vi "fg_ROI Management.vi"(5 "Function":T4, 8 "error in (no error)":errorcluster, 9 "ROI management Input cluster":T2, 10 "Offsets cluster":T1, 11 "Reuse last composite ID":bool) -> (0 "error out":errorcluster, 1 "Last composite ID":i32, 2 "Number of ROI":i32, 3 "ROI Setup":T5[](array[typedef]) {"ROI group ID" format="%#_6f"; "Laser Power (%)" format="%#_6f"; "Zoom" format="%#_6f"; "Frame Size" format="%#_6f"; "Number of lines" format="%#_6f"; "Composite ID" format="%#_6f"; "Angle (deg)" format="%#_6f"; "ROI Time (ns)" format="%#_6f"; "ROI ID" format="%#_6f"; "Pixels in ROI" format="%#_6f"; "ROI index" format="%#_6f"; "Z stop" format="%#_6f"; "Y stop" format="%#_6f"; "X stop" format="%#_6f"; "Z start" format="%#_6f"; "X start" format="%#_6f"; "Y start" format="%#_6f"}, 6 "Exceeded limit number of lines":bool)   [LabVIEW 2013]
uses:
  Visualisation/Functional Imaging Viewer/Typedefs/ROI parameters data type.ctl
  Typedefs/ROI management FG states.ctl
  Typedefs/ROI management Input cluster.ctl
  Typedefs/ROI ID Enum.ctl
  Typedefs/Offsets cluster.ctl
  Global Variables/General Globals.vi
  ROI Entry screen/Globals/gl_ROI Entry UI globals.vi
panel:
  out "Number of lines left":i32
  # "X Start\nY Start\nX Stop\nY Stop"
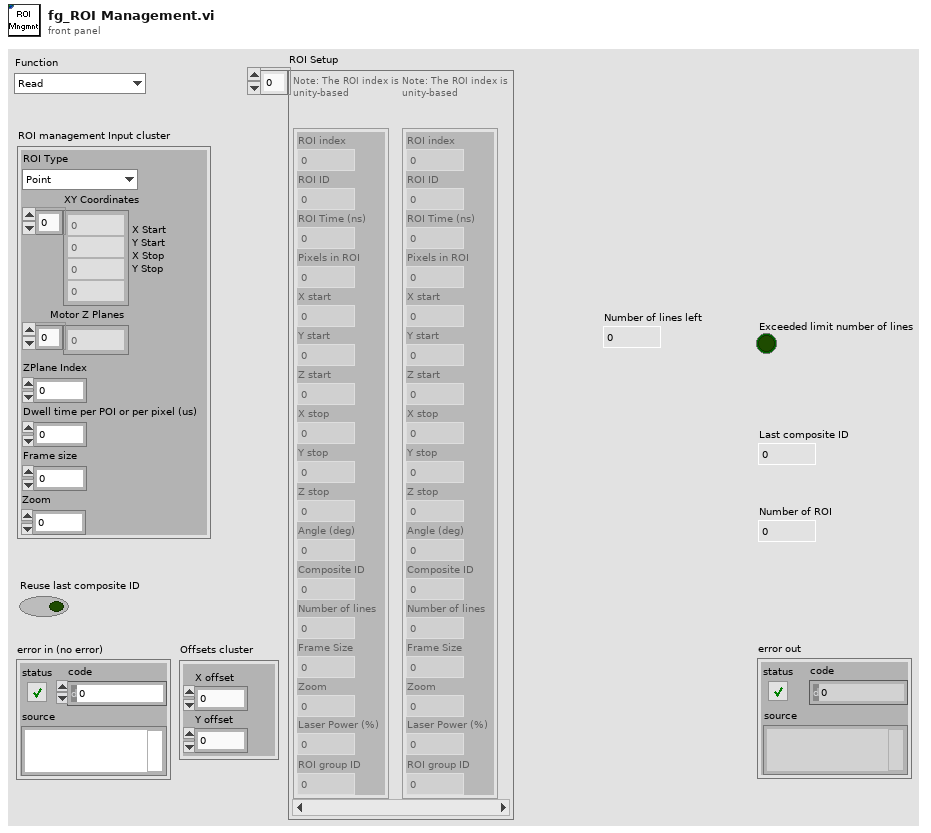
[diagram p1: front panel]
types:
  T1 = typedef "Offsets cluster.ctl" = cluster{"X offset":i8, "Y offset":i8}
  T2 = typedef "ROI management Input cluster.ctl" = cluster{"ROI Type":T3, "XY Coordinates":i32[], "Motor Z Planes":dbl[], "ZPlane Index":i32, "Dwell time per POI or per pixel (us)":dbl, "Frame size":i32, "Zoom":dbl}
  T3 = typedef "ROI ID Enum.ctl" = enum16{"Point", "MiniScan", "Comp. MiniScan", "Rectangle", "Comp. volume", "Arb. plane point"}
  T4 = typedef "ROI management FG states.ctl" = enum16{"Read", "Write", "Clear Last", "Clear All", "Update ROIs time", "Reload last ROI set", "Offset all ROI", "Offset visible ROI"}
  T5 = typedef "ROI parameters data type.ctl" = cluster{"ROI index":dbl, "ROI ID":dbl, "ROI Time (ns)":dbl, "Pixels in ROI":dbl, "X start":dbl, "Y start":dbl, "Z start":dbl, "X stop":dbl, "Y stop":dbl, "Z stop":dbl, "Angle (deg)":dbl, "Composite ID":dbl, "Number of lines":dbl, "Frame Size":dbl, "Zoom":dbl, "Laser Power (%)":dbl, "ROI group ID":dbl}
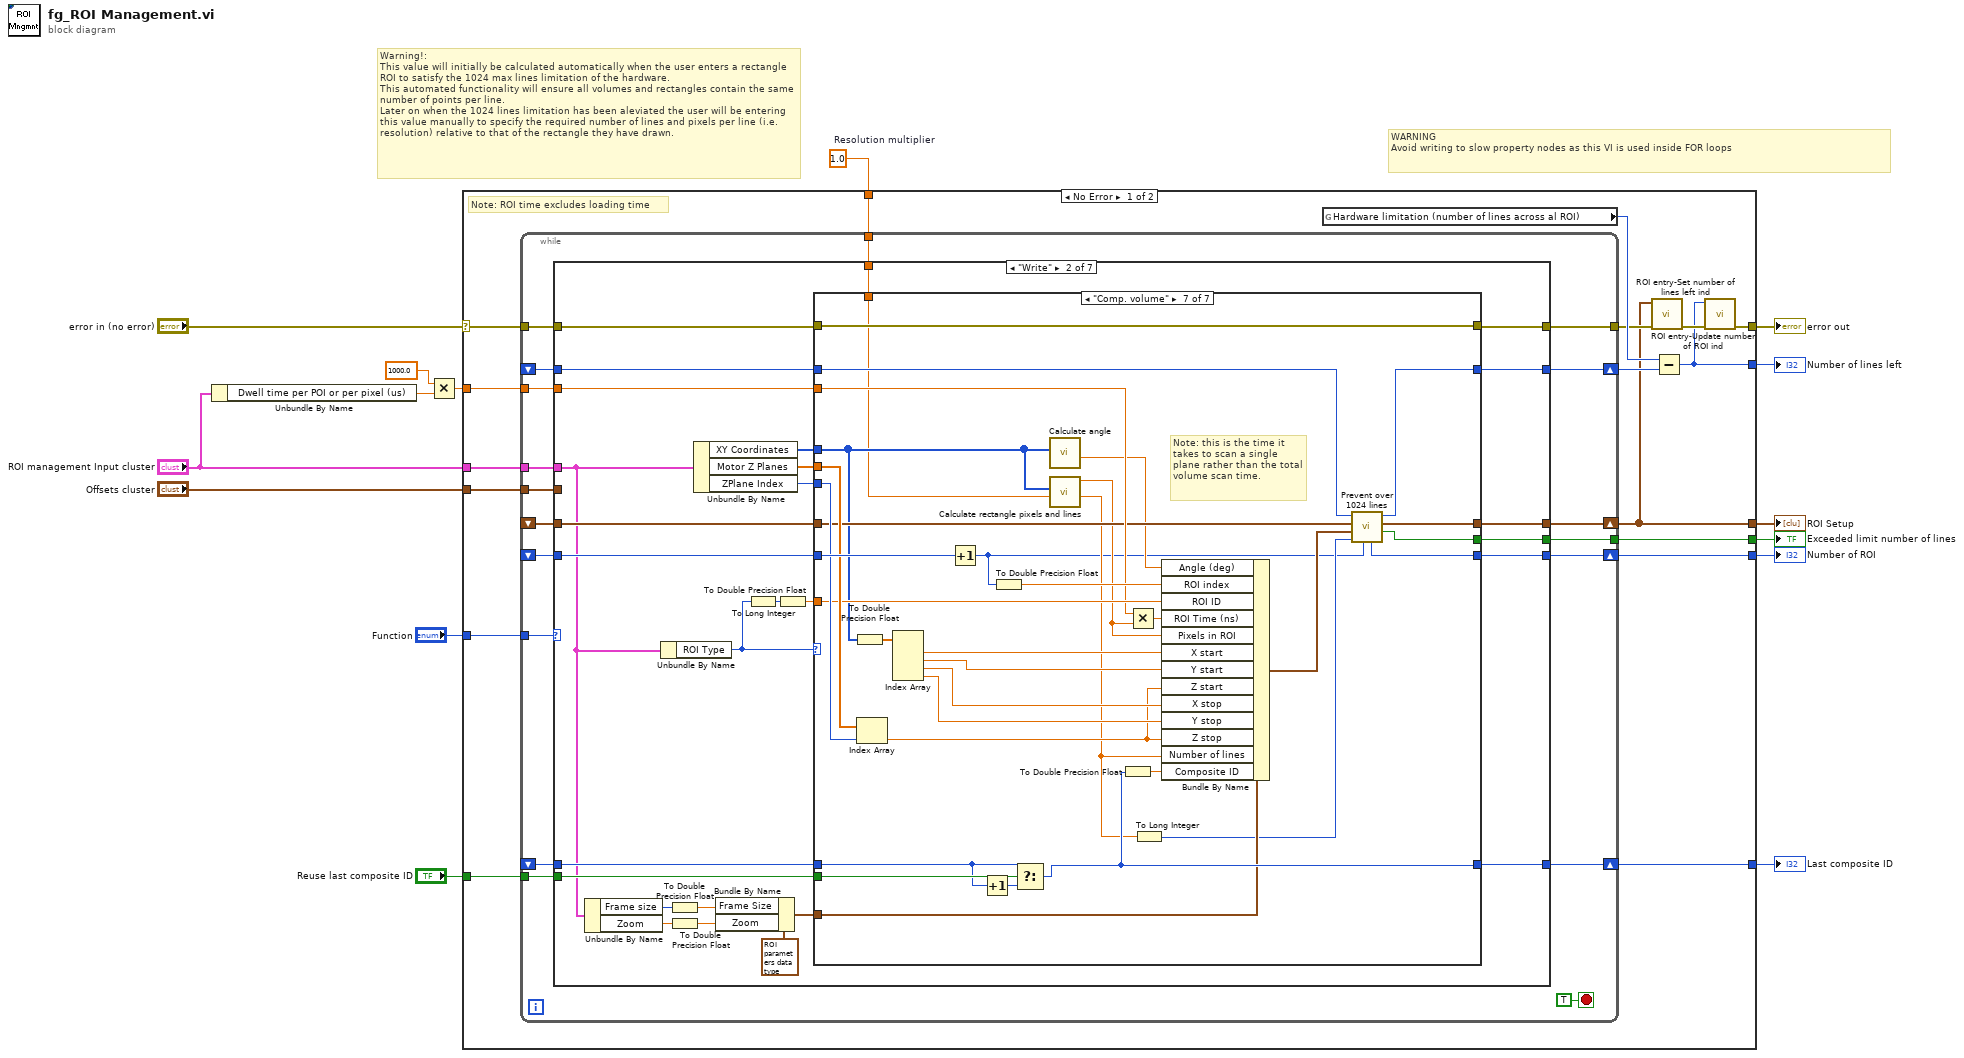
[diagram p0: block diagram]
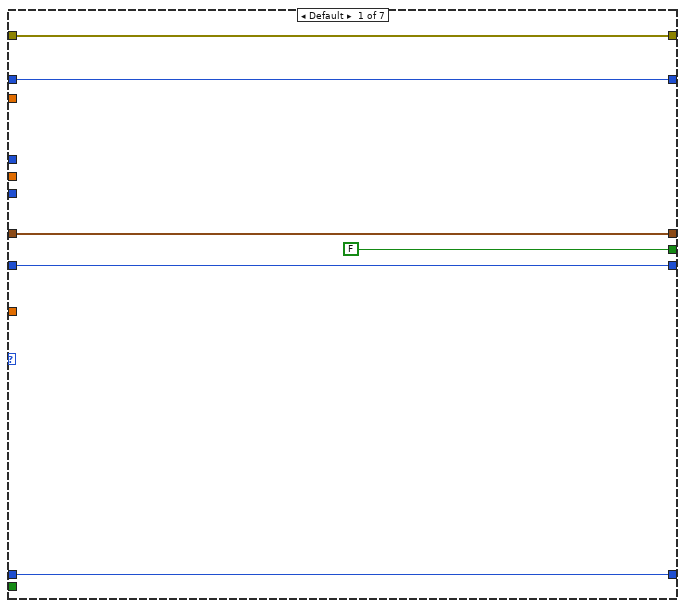
[diagram p3: hidden frame]
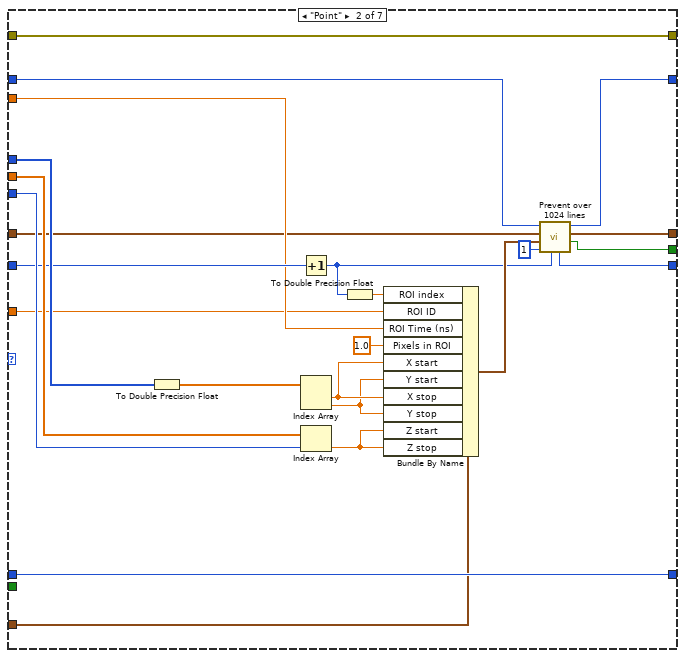
[diagram p4: hidden frame]
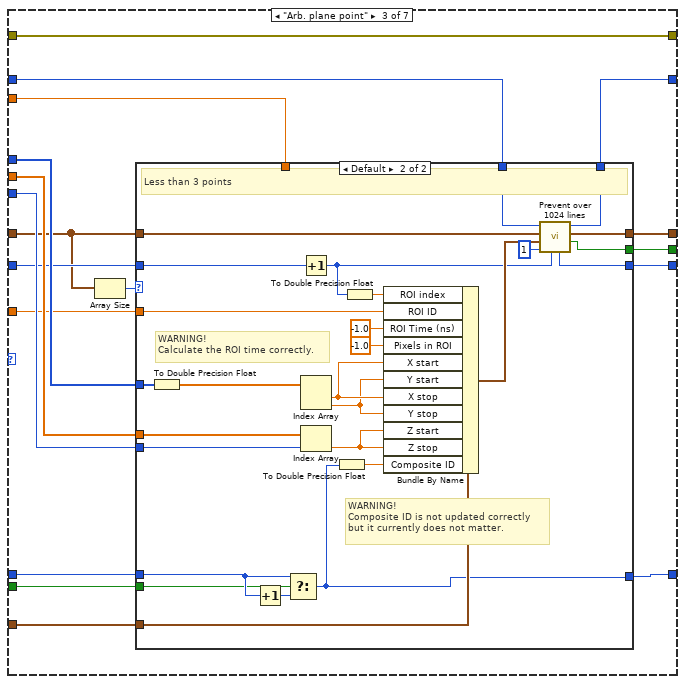
[diagram p5: hidden frame]
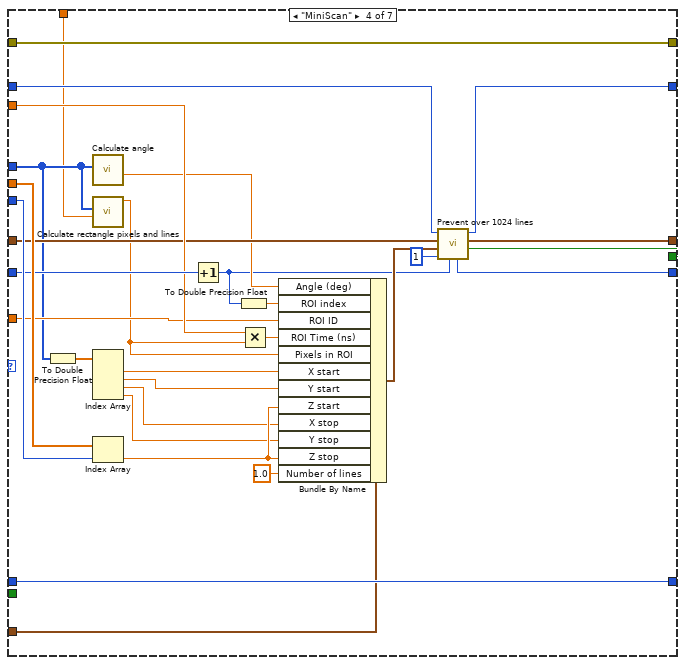
[diagram p7: hidden frame]
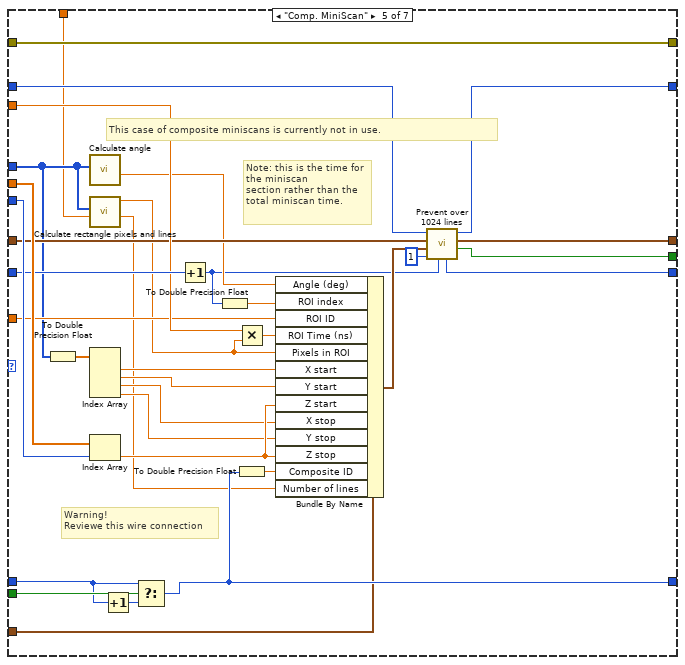
[diagram p8: hidden frame]
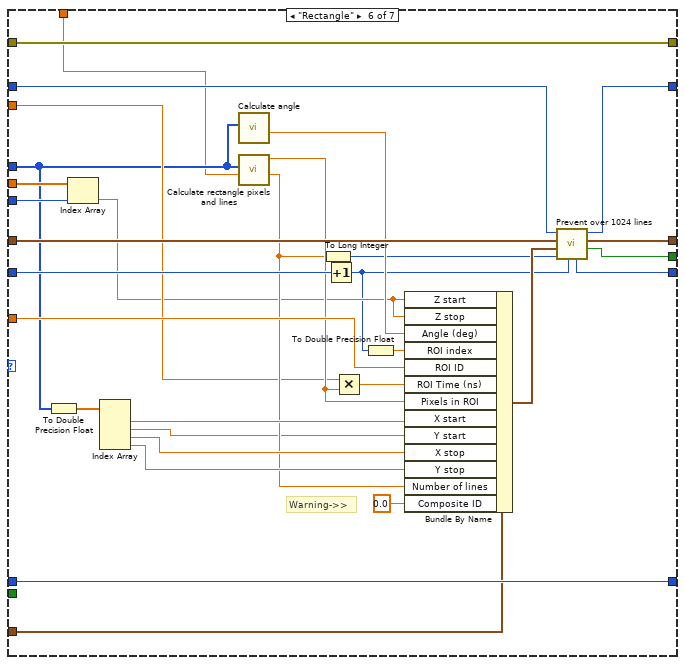
[diagram p9: hidden frame]
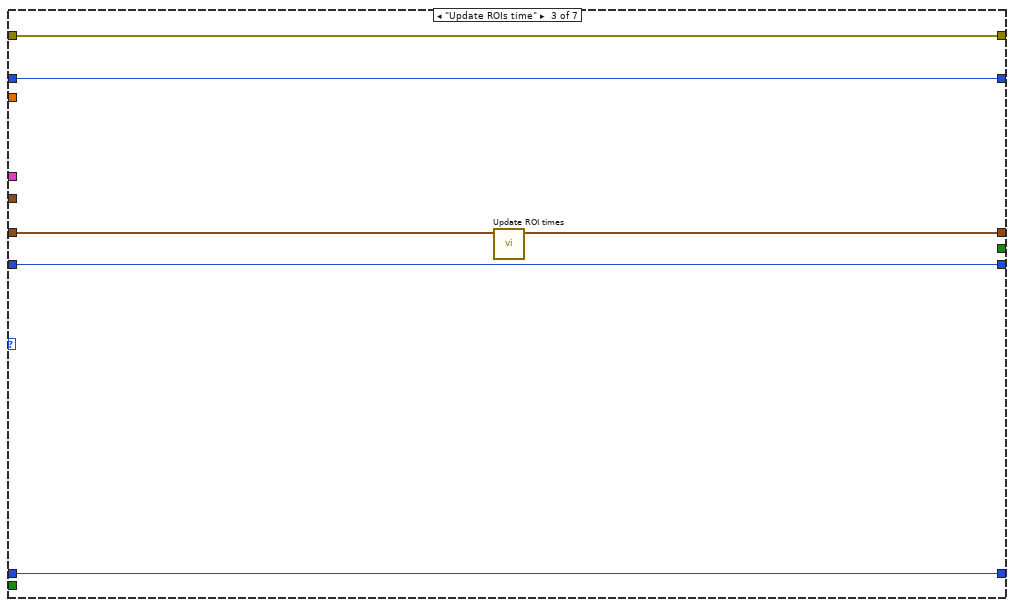
[diagram p10: hidden frame]
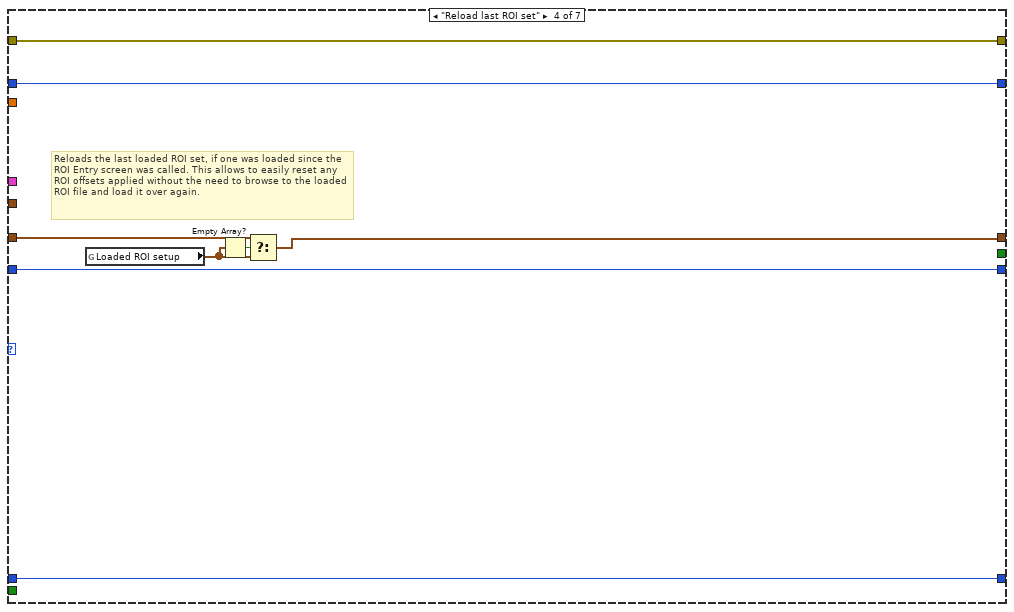
[diagram p11: hidden frame]
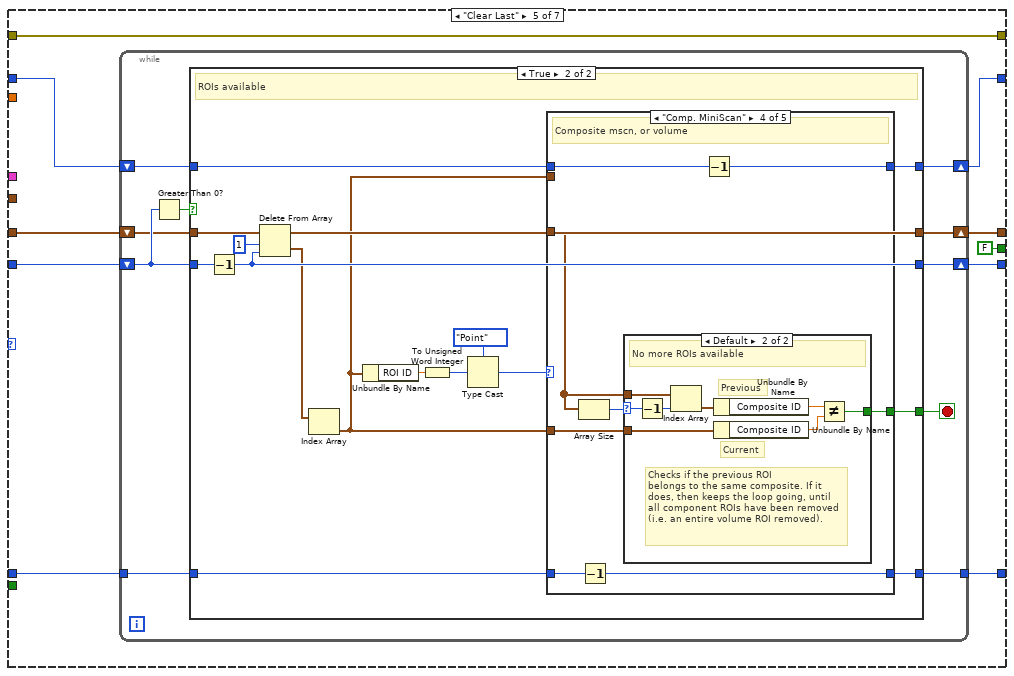
[diagram p12: hidden frame]
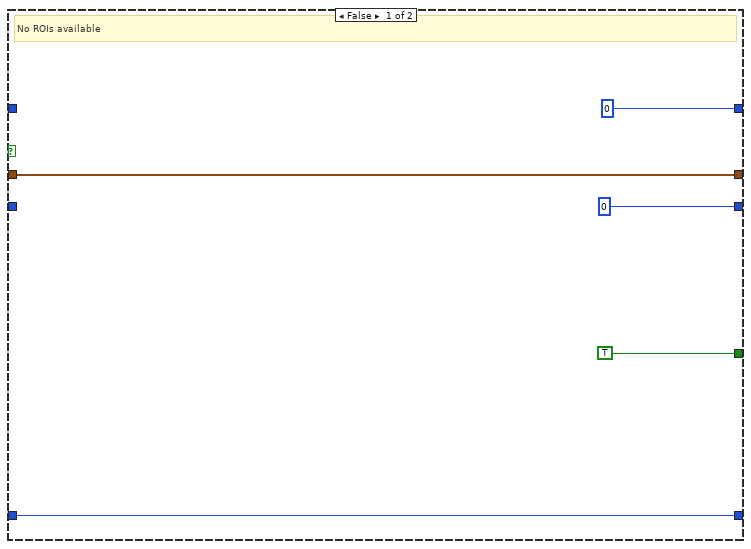
[diagram p13: hidden frame]
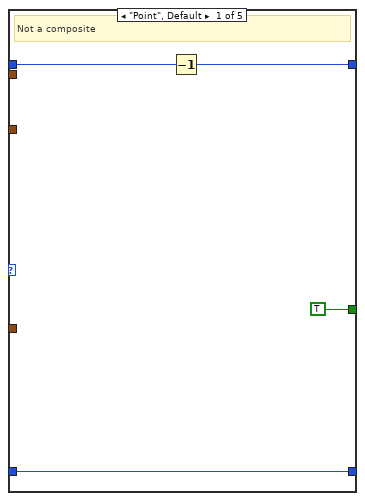
[diagram p14: hidden frame]
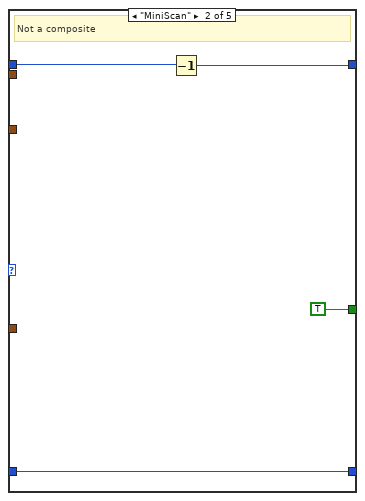
[diagram p15: hidden frame]
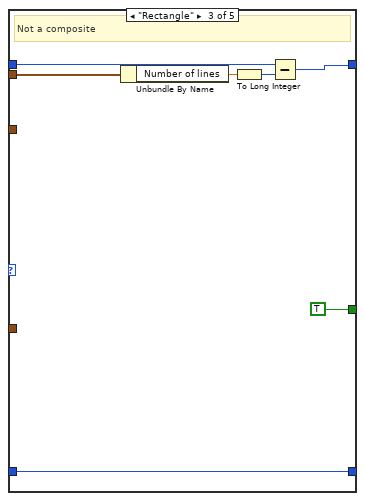
[diagram p16: hidden frame]
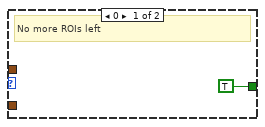
[diagram p17: hidden frame]
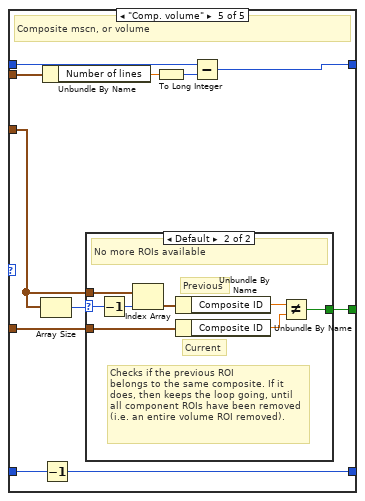
[diagram p18: hidden frame]
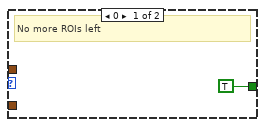
[diagram p19: hidden frame]
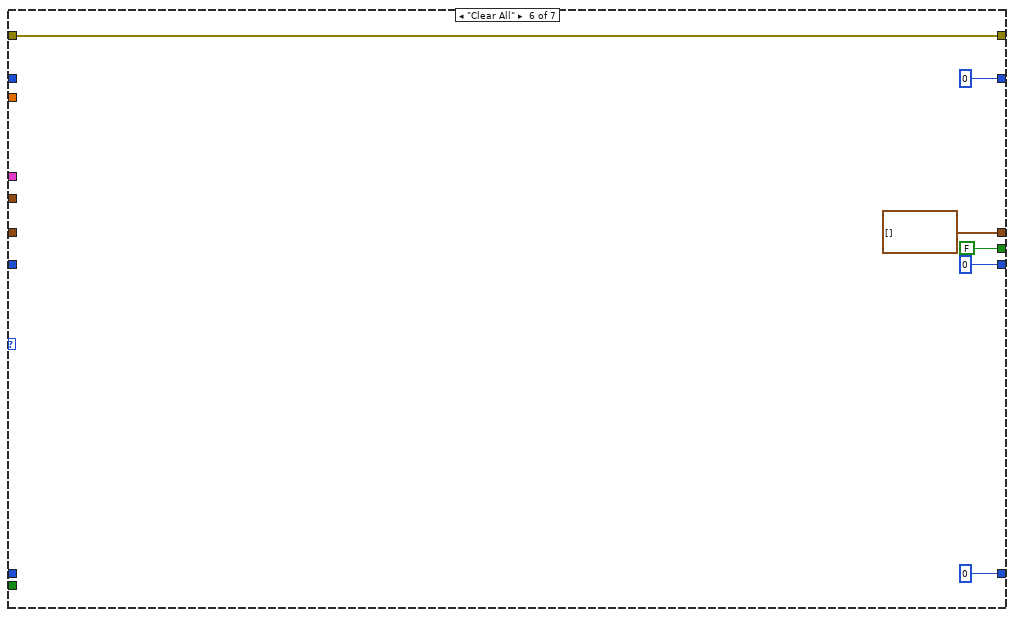
[diagram p20: hidden frame]
diagram:
  w5 = 1.0  # Resolution multiplier
  # "WARNING\nAvoid writing to slow property nodes as this VI is used inside FOR loops"
  # "Warning!:\nThis value will initially be calculated automatically when the user enters a rectangle ROI to satisfy the 1024 max lines limitation of the hardware.\nThis automated functionality will ensure all volumes and rectangles contain the same number of points per line.\nLater on when the 1024 lines limitation has been aleviated the user will be entering this value manually to specify the required number of lines and pixels per line (i.e. resolution) relative to that of the rectangle they have drawn."
  n1 = Unbundle By Name("ROI management Input cluster") -> ("Dwell time per POI or per pixel (us)"=w6:dbl)
  n2 = Multiply(x=1000.0, y=w6) -> (x*y=w11:dbl)
  n3 = case shown="No Error" "error in (no error)" {
    selector: "error in (no error)" -> [w32 w412]
    tunnel: [w18 w412] -> w12
    tunnel: [w20 _] -> w14
    tunnel: w11 -> [w31 _]
    tunnel: "Function" -> [w30 _]
    tunnel: [w29 _] -> w9
    tunnel: [w28 _] -> w8
    tunnel: "Reuse last composite ID" -> [w27 _]
    tunnel: "ROI management Input cluster" -> [w26 _]
    tunnel: w5 -> [w25 _]
    tunnel: [w17 _] -> w3
    tunnel: [w22 _] -> w2
    tunnel: "Offsets cluster" -> [w16 _]
    frame No Error {
      # "Note: ROI time excludes loading time"
      n4 = while {
        tunnel: w32 -> [w50]
        tunnel: [w49] -> w21
        shift-right: [w48] -> w20
        shift-left: _ -> [w46]
        tunnel: w31 -> [w47]
        shift-right: [w45] -> w29
        shift-left: _ -> [w44]
        tunnel: w30 -> [w43]
        shift-right: [w40] -> w28
        shift-left: _ -> [w41]
        tunnel: w27 -> [w39]
        tunnel: w26 -> [w38]
        shift-right: [w37] -> w24
        shift-left: _ -> [w36]
        tunnel: w25 -> [w35]
        tunnel: [w34] -> w22
        tunnel: w16 -> [w33]
        stop <- TRUE stop-if-true
        n5 = case shown="\"Write\"" w43 {
          selector: w43 -> [_ _ _ _ _ _ w404]
          tunnel: w50 -> [w53 w82 w294 w303 w312 w402 w410]
          tunnel: [w53 w81 w294 w303 w312 w402 w410] -> w49
          tunnel: [w55 w80 w296 w298 w313 T5[] [] w405] -> w48
          tunnel: w47 -> [_ w79 _ _ _ _ _]
          tunnel: w46 -> [w55 w78 w292 w299 w308 _ w408]
          tunnel: [w54 w77 w295 w304 w314 0 w411] -> w45
          tunnel: w44 -> [w54 w76 w295 w304 w309 _ w411]
          tunnel: w41 -> [w52 w72 w291 w301 w311 _ w407]
          tunnel: [w52 w73 w291 w301 w310 0 ("Last composite ID") w407] -> w40
          tunnel: w39 -> [_ w71 _ _ _ _ _]
          tunnel: w38 -> [_ w65 _ _ _ _ _]
          tunnel: [w51 w58 w293 w302 w305 0 w409] -> w37
          tunnel: w36 -> [w51 w60 w293 w302 w307 _ w409]
          tunnel: w35 -> [_ w59 _ _ _ _ _]
          tunnel: [_ w57 _ _ FALSE ("Exceeded 1024 lines") FALSE ("Exceeded 1024 lines") _] -> w34
          tunnel: w33 -> [_ _ _ _ _ _ w406]
          frame "Read", Default {
          }
          frame "Write" {
            n6 = Unbundle By Name(w65) -> ("Frame size"=w66:i32, "Zoom"=w62:dbl)
            n7 = Unbundle By Name(w65) -> ("ROI Type"=w67:T3)
            n8 = To Double Precision Float(number=w66) -> (double precision float=w64:dbl)
            n9 = To Double Precision Float(number=w62) -> (double precision float=w61:dbl)
            n10 = Unbundle By Name(w65) -> ("XY Coordinates"=w70:i32[], "Motor Z Planes"=w69:dbl[], "ZPlane Index"=w68:i32)
            n11 = Bundle By Name(cluster=T5 {"ROI index"=0.0, "ROI ID"=0.0, "ROI Time (ns)"=0.0, "Pixels in ROI"=0.0, "X start"=0.0, "Y start"=0.0, "Z start"=0.0, "X stop"=0.0, "Y stop"=0.0, "Z stop"=0.0, "Angle (deg)"=0.0, "Composite ID"=0.0, "Number of lines"=0.0, "Frame Size"=0.0, "Zoom"=0.0, "Laser Power (%)"=0.0, "ROI group ID"=0.0} ("X-Y-Z coordinates"), "Frame Size"=w64, "Zoom"=w61) -> (w63:T5)
            n12 = To Long Integer(number=w67) -> (32bit integer=w75:i32)
            n13 = To Double Precision Float(number=w75) -> (double precision float=w74:dbl)
            n14 = case shown="\"Comp. volume\"" w67 {
              tunnel: w70 -> [_ w109 w127 w169 w198 w233 w263]
              tunnel: w69 -> [_ w111 w129 w190 w224 w253 w283]
              tunnel: w82 -> [w86 w112 w130 w191 w225 w256 w290]
              tunnel: [w86 w112 w130 w191 w225 w256 w290] -> w81
              tunnel: w68 -> [_ w110 w128 w189 w223 w252 w282]
              tunnel: [w88 w97 w123 w174 w203 w244 w268] -> w80
              tunnel: w79 -> [_ w105 w125 w184 w218 w234 w277]
              tunnel: w78 -> [w88 w98 w119 w176 w205 w246 w270]
              tunnel: w76 -> [w87 w107 w126 w188 w222 w255 w289]
              tunnel: [w87 w89 w117 w162 w192 w226 w257] -> w77
              tunnel: w74 -> [_ w101 w113 w180 w212 w251 w280]
              tunnel: [w85 w100 w114 w179 w208 w248 w272] -> w73
              tunnel: w72 -> [w85 w100 w116 w179 w207 w248 w274]
              tunnel: w71 -> [_ _ w115 _ w209 _ w275]
              tunnel: w63 -> [_ w99 w124 w178 w206 w247 w271]
              tunnel: [w84 w96 w122 w171 w202 w243 w267] -> w58
              tunnel: w60 -> [w84 w95 w121 w172 w200 w242 w266]
              tunnel: w59 -> [_ _ _ w165 w195 w228 w259]
              tunnel: [FALSE ("Exceeded 1024 lines") w93 w120 w170 w199 w241 w264] -> w57
              frame Default {
              }
              frame "Point" {
                n15 = To Double Precision Float(number=w109) -> (double precision float=w103:dbl[])
                n16 = Increment(x=w107) -> (x+1=w90:i32)
                n17 = Index Array(array=w103) -> (element #1=w104:dbl, element #2=w92:dbl)  [unwired: 2 in]
                n18 = Index Array(array=w111, index=w110) -> (element=w91:dbl)
                n19 = To Double Precision Float(number=w90) -> (double precision float=w102:dbl)
                n20 = Bundle By Name(cluster=w99, "ROI index"=w102, "ROI ID"=w101, "ROI Time (ns)"=w105, "Pixels in ROI"=1.0 ("#Pixels"), "X start"=w104, "Y start"=w92, "X stop"=w104, "Y stop"=w92, "Z start"=w91, "Z stop"=w91) -> (w108:T5)
                n21 = call "Prevent over 1024 lines.vi"("Number of ROI"=w90, "New number of lines to be added (1)"=1, "X-Y-Z coordinates"=w108, "Array in"=w98, "Existing number of lines across all ROI"=w95) -> ("Exceeded 1024 lines"=w93:bool, "Array out"=w97:T5[], "Resulting number of lines across all ROI"=w96:i32, "Number of ROI"=w89:i32)  [unwired: 2 in, 1 out]
              }
              frame "Arb. plane point" {
                n22 = Array Size(array=w119) -> (size(s)=w118:i32)
                n23 = case shown="Default" w118 {
                  selector: w118 -> [w132 _]
                  tunnel: w129 -> [_ w161]
                  tunnel: w128 -> [_ w160]
                  tunnel: w127 -> [_ w159]
                  tunnel: w126 -> [_ w157]
                  tunnel: w125 -> [_ _]
                  tunnel: w124 -> [_ w152]
                  tunnel: [w133 w151] -> w123
                  tunnel: [w134 w150] -> w122
                  tunnel: w121 -> [w134 w149]
                  tunnel: [_ w147] -> w120
                  tunnel: w119 -> [w133 w144]
                  tunnel: [w132 w135] -> w117
                  tunnel: w116 -> [w131 w142]
                  tunnel: w115 -> [_ w141]
                  tunnel: [w131 w139] -> w114
                  tunnel: w113 -> [_ w138]
                  frame 3.. {
                    # "3 points (or more) already entered"
                  }
                  frame Default {
                    # "WARNING!\nComposite ID is not updated correctly\nbut it currently does not matter."
                    # "WARNING!\nCalculate the ROI time correctly."
                    # "Less than 3 points"
                    n24 = To Double Precision Float(number=w159) -> (double precision float=w154:dbl[])
                    n25 = Increment(x=w142) -> (x+1=w143:i32)
                    n26 = Select(t=w142, s=w141, f=w143) -> (s? t:f=w139:i32)
                    n27 = Increment(x=w157) -> (x+1=w136:i32)
                    n28 = Index Array(array=w154) -> (element #1=w155:dbl, element #2=w146:dbl)  [unwired: 2 in]
                    n29 = Index Array(array=w161, index=w160) -> (element=w145:dbl)
                    n30 = To Double Precision Float(number=w139) -> (double precision float=w140:dbl)
                    n31 = To Double Precision Float(number=w136) -> (double precision float=w153:dbl)
                    n32 = Bundle By Name(cluster=w152, "ROI index"=w153, "ROI ID"=w138, "ROI Time (ns)"=-1.0, "Pixels in ROI"=-1.0 ("#Pixels"), "X start"=w155, "Y start"=w146, "X stop"=w155, "Y stop"=w146, "Z start"=w145, "Z stop"=w145, "Composite ID"=w140) -> (w158:T5)
                    n33 = call "Prevent over 1024 lines.vi"("Number of ROI"=w136, "New number of lines to be added (1)"=1, "X-Y-Z coordinates"=w158, "Array in"=w144, "Existing number of lines across all ROI"=w149) -> ("Exceeded 1024 lines"=w147:bool, "Array out"=w151:T5[], "Resulting number of lines across all ROI"=w150:i32, "Number of ROI"=w135:i32)  [unwired: 2 in, 1 out]
                  }
                }
              }
              frame "MiniScan" {
                n34 = To Double Precision Float(number=w169) -> (double precision float=w185:dbl[])
                n35 = call "Calculate angle.vi"("XY Coordinates"=w169) -> ("Angle (deg)"=w167:dbl)  [unwired: 10 in]
                n36 = call "Calculate rectangle pixels and lines.vi"("Resolution multiplier"=w165, "XY Coordinates (zero based)"=w169) -> ("Pixels in ROI"=w168:dbl)  [unwired: 8 in, 1 out]
                n37 = Index Array(array=w185) -> (element #1=w166:dbl, element #2=w186:dbl, element #3=w177:dbl, element #4=w181:dbl)  [unwired: 4 in]
                n38 = Index Array(array=w190, index=w189) -> (element=w187:dbl)
                n39 = Increment(x=w188) -> (x+1=w163:i32)
                n40 = To Double Precision Float(number=w163) -> (double precision float=w183:dbl)
                n41 = Multiply(x=w184, y=w168) -> (x*y=w182:dbl)
                n42 = Bundle By Name(cluster=w178, "Angle (deg)"=w167, "ROI index"=w183, "ROI ID"=w180, "ROI Time (ns)"=w182, "Pixels in ROI"=w168, "X start"=w166, "Y start"=w186, "Z start"=w187, "X stop"=w177, "Y stop"=w181, "Z stop"=w187, "Number of lines"=1.0) -> (w175:T5)
                n43 = call "Prevent over 1024 lines.vi"("Number of ROI"=w163, "New number of lines to be added (1)"=1, "X-Y-Z coordinates"=w175, "Array in"=w176, "Existing number of lines across all ROI"=w172) -> ("Exceeded 1024 lines"=w170:bool, "Array out"=w174:T5[], "Resulting number of lines across all ROI"=w171:i32, "Number of ROI"=w162:i32)  [unwired: 2 in, 1 out]
              }
              frame "Comp. MiniScan" {
                # "This case of composite miniscans is currently not in use."
                # "Warning!\nReviewe this wire connection"
                # "Note: this is the time for the miniscan\nsection rather than the total miniscan time."
                n44 = To Double Precision Float(number=w198) -> (double precision float=w219:dbl[])
                n45 = call "Calculate angle.vi"("XY Coordinates"=w198) -> ("Angle (deg)"=w196:dbl)  [unwired: 10 in]
                n46 = call "Calculate rectangle pixels and lines.vi"("Resolution multiplier"=w195, "XY Coordinates (zero based)"=w198) -> ("Number of lines (scaled)"=w194:dbl, "Pixels in ROI"=w197:dbl)  [unwired: 8 in]
                n47 = Index Array(array=w219) -> (element #1=w215:dbl, element #2=w220:dbl, element #3=w214:dbl, element #4=w213:dbl)  [unwired: 4 in]
                n48 = Index Array(array=w224, index=w223) -> (element=w221:dbl)
                n49 = Increment(x=w207) -> (x+1=w210:i32)
                n50 = Select(t=w207, s=w209, f=w210) -> (s? t:f=w208:i32)
                n51 = Increment(x=w222) -> (x+1=w193:i32)
                n52 = To Double Precision Float(number=w193) -> (double precision float=w217:dbl)
                n53 = Multiply(x=w218, y=w197) -> (x*y=w216:dbl)
                n54 = To Double Precision Float(number=w208) -> (double precision float=w211:dbl)
                n55 = Bundle By Name(cluster=w206, "Angle (deg)"=w196, "ROI index"=w217, "ROI ID"=w212, "ROI Time (ns)"=w216, "Pixels in ROI"=w197, "X start"=w215, "Y start"=w220, "Z start"=w221, "X stop"=w214, "Y stop"=w213, "Z stop"=w221, "Composite ID"=w211, "Number of lines"=w194) -> (w204:T5)
                n56 = call "Prevent over 1024 lines.vi"("Number of ROI"=w193, "New number of lines to be added (1)"=1, "X-Y-Z coordinates"=w204, "Array in"=w205, "Existing number of lines across all ROI"=w200) -> ("Exceeded 1024 lines"=w199:bool, "Array out"=w203:T5[], "Resulting number of lines across all ROI"=w202:i32, "Number of ROI"=w192:i32)  [unwired: 2 in, 1 out]
              }
              frame "Rectangle" {
                # "Warning->>"
                n57 = To Double Precision Float(number=w233) -> (double precision float=w254:dbl[])
                n58 = Index Array(array=w253, index=w252) -> (element=w229:dbl)
                n59 = Index Array(array=w254) -> (element #1=w240:dbl, element #2=w235:dbl, element #3=w239:dbl, element #4=w238:dbl)  [unwired: 4 in]
                n60 = call "Calculate angle.vi"("XY Coordinates"=w233) -> ("Angle (deg)"=w232:dbl)  [unwired: 10 in]
                n61 = call "Calculate rectangle pixels and lines.vi"("Resolution multiplier"=w228, "XY Coordinates (zero based)"=w233) -> ("Number of lines (scaled)"=w236:dbl, "Pixels in ROI"=w237:dbl)  [unwired: 8 in]
                n62 = To Long Integer(number=w236) -> (32bit integer=w230:i32)
                n63 = Increment(x=w255) -> (x+1=w227:i32)
                n64 = Multiply(x=w234, y=w237) -> (x*y=w249:dbl)
                n65 = To Double Precision Float(number=w227) -> (double precision float=w250:dbl)
                n66 = Bundle By Name(cluster=w247, "Z start"=w229, "Z stop"=w229, "Angle (deg)"=w232, "ROI index"=w250, "ROI ID"=w251, "ROI Time (ns)"=w249, "Pixels in ROI"=w237, "X start"=w240, "Y start"=w235, "X stop"=w239, "Y stop"=w238, "Number of lines"=w236, "Composite ID"=0.0) -> (w245:T5)
                n67 = call "Prevent over 1024 lines.vi"("Number of ROI"=w227, "New number of lines to be added (1)"=w230, "X-Y-Z coordinates"=w245, "Array in"=w246, "Existing number of lines across all ROI"=w242) -> ("Exceeded 1024 lines"=w241:bool, "Array out"=w244:T5[], "Resulting number of lines across all ROI"=w243:i32, "Number of ROI"=w226:i32)  [unwired: 2 in, 1 out]
              }
              frame "Comp. volume" {
                # "Note: this is the time it takes to scan a single plane rather than the total volume scan time."
                n68 = To Double Precision Float(number=w263) -> (double precision float=w284:dbl[])
                n69 = Index Array(array=w283, index=w282) -> (element=w281:dbl)
                n70 = Index Array(array=w284) -> (element #1=w285:dbl, element #2=w288:dbl, element #3=w287:dbl, element #4=w286:dbl)  [unwired: 4 in]
                n71 = Increment(x=w289) -> (x+1=w258:i32)
                n72 = Increment(x=w274) -> (x+1=w273:i32)
                n73 = To Double Precision Float(number=w258) -> (double precision float=w279:dbl)
                n74 = Select(t=w274, s=w275, f=w273) -> (s? t:f=w272:i32)
                n75 = call "Calculate angle.vi"("XY Coordinates"=w263) -> ("Angle (deg)"=w262:dbl)  [unwired: 10 in]
                n76 = call "Calculate rectangle pixels and lines.vi"("Resolution multiplier"=w259, "XY Coordinates (zero based)"=w263) -> ("Number of lines (scaled)"=w260:dbl, "Pixels in ROI"=w261:dbl)  [unwired: 8 in]
                n77 = To Double Precision Float(number=w272) -> (double precision float=w276:dbl)
                n78 = Multiply(x=w277, y=w261) -> (x*y=w278:dbl)
                n79 = To Long Integer(number=w260) -> (32bit integer=w265:i32)
                n80 = Bundle By Name(cluster=w271, "Angle (deg)"=w262, "ROI index"=w279, "ROI ID"=w280, "ROI Time (ns)"=w278, "Pixels in ROI"=w261, "X start"=w285, "Y start"=w288, "Z start"=w281, "X stop"=w287, "Y stop"=w286, "Z stop"=w281, "Number of lines"=w260, "Composite ID"=w276) -> (w269:T5)
                n81 = call "Prevent over 1024 lines.vi"("Number of ROI"=w258, "New number of lines to be added (1)"=w265, "X-Y-Z coordinates"=w269, "Array in"=w270, "Existing number of lines across all ROI"=w266) -> ("Exceeded 1024 lines"=w264:bool, "Array out"=w268:T5[], "Resulting number of lines across all ROI"=w267:i32, "Number of ROI"=w257:i32)  [unwired: 2 in, 1 out]
              }
            }
          }
          frame "Update ROIs time" {
            n82 = call "Update ROI times.vi"("ROI setup in"=w292) -> ("ROI setup out"=w296:T5[])  [unwired: 10 in]
          }
          frame "Reload last ROI set" {
            # "Reloads the last loaded ROI set, if one was loaded since the ROI Entry screen was called. This allows to easily reset any ROI offsets applied without the need to browse to the loaded ROI file and load it over again."
            n83 = global read "gl_ROI Entry UI globals.vi" "Loaded ROI setup"() -> (w297:T5[])
            n84 = Empty Array?(array=w297) -> (empty?=w300:bool)
            n85 = Select(t=w299, s=w300, f=w297) -> (s? t:f=w298:T5[])
          }
          frame "Clear Last" {
            n86 = while {
              tunnel: w311 -> [w321]
              tunnel: [w320] -> w310
              shift-right: [w324] -> w314
              shift-left: w309 -> [w318]
              shift-right: [w323] -> w313
              shift-left: w308 -> [w317]
              shift-right: [w315] -> w305
              shift-left: w307 -> [w316]
              stop <- w319 stop-if-true
              n87 = Greater Than 0?(x=w318) -> (x > 0?=w322:bool)
              n88 = case shown="True" w322 {
                tunnel: [0 w342] -> w324
                tunnel: w317 -> [w328 w345]
                tunnel: [w328 w336] -> w323
                tunnel: w318 -> [_ w344]
                tunnel: w321 -> [w327 w339]
                tunnel: [w327 w338] -> w320
                tunnel: [TRUE w337] -> w319
                tunnel: w316 -> [_ w335]
                tunnel: [0 w334] -> w315
                frame False {
                  # "No ROIs available"
                }
                frame True {
                  # "ROIs available"
                  n89 = Decrement(x=w344) -> (x-1=w342:i32)
                  n90 = Delete From Array "Delete From Array"(array=w345, length=1, index=w342) -> (deleted portion=w341:T5[], array with subset deleted=w336:T5[])
                  n91 = Index Array(array=w341) -> (element=w330:T5)  [unwired: 1 in]
                  n92 = Unbundle By Name(w330) -> ("ROI ID"=w340:dbl)
                  n93 = To Unsigned Word Integer(number=w340) -> (unsigned 16bit integer=w333:u16)
                  n94 = Type Cast(type=ROI_ID_Enum."Point" ("ROI Type"), x=w333) -> (*(type *) &x=w332:T3)
                  n95 = case shown="\"Comp. MiniScan\"" w332 {
                    tunnel: w339 -> [w349 w353 w360 w368 w388]
                    tunnel: [w349 w353 w360 w367 w387] -> w338
                    tunnel: [TRUE TRUE TRUE w364 w384] -> w337
                    tunnel: w336 -> [_ _ _ w363 w383]
                    tunnel: w330 -> [_ _ _ w366 w386]
                    tunnel: w335 -> [w347 w351 w356 w362 w380]
                    tunnel: [w346 w350 w355 w361 w379] -> w334
                    tunnel: w330 -> [_ _ w354 _ w378]
                    frame "Point", Default {
                      # "Not a composite"
                      n96 = Decrement(x=w347) -> (x-1=w346:i32)
                    }
                    frame "MiniScan" {
                      # "Not a composite"
                      n97 = Decrement(x=w351) -> (x-1=w350:i32)
                    }
                    frame "Rectangle" {
                      # "Not a composite"
                      n98 = Unbundle By Name(w354) -> ("Number of lines"=w357:dbl)
                      n99 = To Long Integer(number=w357) -> (32bit integer=w358:i32)
                      n100 = Subtract(x=w356, y=w358) -> (x-y=w355:i32)
                    }
                    frame "Comp. MiniScan" {
                      # "Composite mscn, or volume"
                      n101 = Array Size(array=w363) -> (size(s)=w365:i32)
                      n102 = Decrement(x=w368) -> (x-1=w367:i32)
                      n103 = case shown="Default" w365 {
                        selector: w365 -> [_ w371]
                        tunnel: w363 -> [_ w377]
                        tunnel: w366 -> [_ w374]
                        tunnel: [TRUE w370] -> w364
                        frame 0 {
                          # "No more ROIs left"
                        }
                        frame Default {
                          # "Checks if the previous ROI \nbelongs to the same composite. If it does, then keeps the loop going, until all component ROIs have been removed (i.e. an entire volume ROI removed)."
                          # "Previous"
                          # "Current"
                          # "No more ROIs available"
                          n104 = Decrement(x=w371) -> (x-1=w376:i32)
                          n105 = Index Array(array=w377, index=w376) -> (element=w375:T5)
                          n106 = Unbundle By Name(w375) -> ("Composite ID"=w373:dbl)
                          n107 = Unbundle By Name(w374) -> ("Composite ID"=w372:dbl)
                          n108 = Not Equal?(x=w373, y=w372) -> (x != y?=w370:bool)
                        }
                      }
                      n109 = Decrement(x=w362) -> (x-1=w361:i32)
                    }
                    frame "Comp. volume" {
                      # "Composite mscn, or volume"
                      n110 = Array Size(array=w383) -> (size(s)=w385:i32)
                      n111 = Decrement(x=w388) -> (x-1=w387:i32)
                      n112 = Unbundle By Name(w378) -> ("Number of lines"=w381:dbl)
                      n113 = case shown="Default" w385 {
                        selector: w385 -> [_ w391]
                        tunnel: w383 -> [_ w397]
                        tunnel: w386 -> [_ w394]
                        tunnel: [TRUE w390] -> w384
                        frame 0 {
                          # "No more ROIs left"
                        }
                        frame Default {
                          # "Checks if the previous ROI \nbelongs to the same composite. If it does, then keeps the loop going, until all component ROIs have been removed (i.e. an entire volume ROI removed)."
                          # "Previous"
                          # "Current"
                          # "No more ROIs available"
                          n114 = Decrement(x=w391) -> (x-1=w396:i32)
                          n115 = Index Array(array=w397, index=w396) -> (element=w395:T5)
                          n116 = Unbundle By Name(w395) -> ("Composite ID"=w393:dbl)
                          n117 = Unbundle By Name(w394) -> ("Composite ID"=w392:dbl)
                          n118 = Not Equal?(x=w393, y=w392) -> (x != y?=w390:bool)
                        }
                      }
                      n119 = To Long Integer(number=w381) -> (32bit integer=w382:i32)
                      n120 = Subtract(x=w380, y=w382) -> (x-y=w379:i32)
                    }
                  }
                }
              }
            }
          }
          frame "Clear All" {
          }
          frame "Offset all ROI", "Offset visible ROI" {
            n121 = call "ROI entry-Offset ROI (core).vi"("Function"=w404, "ROI setup in"=w408, "Offsets cluster in"=w406) -> ("ROI setup"=w405:T5[])  [unwired: 8 in]
          }
        }
      }
      n122 = global read "General Globals.vi" "Hardware limitation (number of lines across al ROI)"() -> (w23:i32)
      n123 = call "ROI entry-Update number of ROI ind.vi"("error in (no error)"=w21, "ROI Setup"=w20) -> ("error out"=w19:errorcluster)  [unwired: 9 in]
      n124 = Subtract(x=w23, y=w24) -> (x-y=w17:i32)
      n125 = call "ROI entry-Set number of lines left ind.vi"("error in (no error)"=w19, "Number of lines left"=w17) -> ("error out"=w18:errorcluster)  [unwired: 9 in]
    }
    frame Error {
    }
  }
  "error out" <- w12
  "ROI Setup" <- w14
  "Number of ROI" <- w9
  "Last composite ID" <- w8
  "Number of lines left" <- w3
  "Exceeded limit number of lines" <- w2
